vi "Simulation Initialize.vi"(0 "simulation configuration":T1={"maxTime"=5.0, "enableVisualization"=TRUE, "statechart"=path "iRobot Navigation State Machine.vi", "environment"=path "iRobot Navigation State Machine.vi", "record"=path "Simulation Record.xml", "autograde?"=TRUE, "interactive?"=FALSE, "feedback mode"=enum."debug navigation"}, 2 "Statechart display":refnum<vi>, 3 "Simulator display":refnum<vi>, 11 "Error In":errorcluster) -> (4 "simulator":T3={"configuration"={"maxTime"=5.0, "enableVisualization"=TRUE, "statechart"=path "iRobot Navigation State Machine.vi", "environment"=path "iRobot Navigation State Machine.vi", "record"=path "Simulation Record.xml", "autograde?"=TRUE, "interactive?"=FALSE, "feedback mode"=enum."debug navigation"}, "Bump Sensors"=[], "Distance Sensors"=[], "Accelerometer"=refnum, "Wall Sensor"=refnum, "Statechart\ndisplay"=refnum, "Body"=refnum, "Left Motor"=refnum, "Right Motor"=refnum, "first step?"=FALSE}, 15 "Error Out":errorcluster)   [LabVIEW 2013]
uses:
  Simulator.ctl
  <instrlib>/DC Motor Controller/HAIOL/DC Motor Controller.lvclass
  CyberSim interface/Simulation Configuration.ctl
  autograder/feedbackMode.ctl
  <vilib>/robotics/Simulator/Engine/ctl/Simulation Mode.ctl
  <vilib>/robotics/Simulator/Engine/ctl/Step Mode.ctl
  Simulation Trace Operation.ctl
  Simulation Call Statechart Operation.ctl
  <vilib>/robotics/Simulator/NI_Robotics_Simulator.lvlib
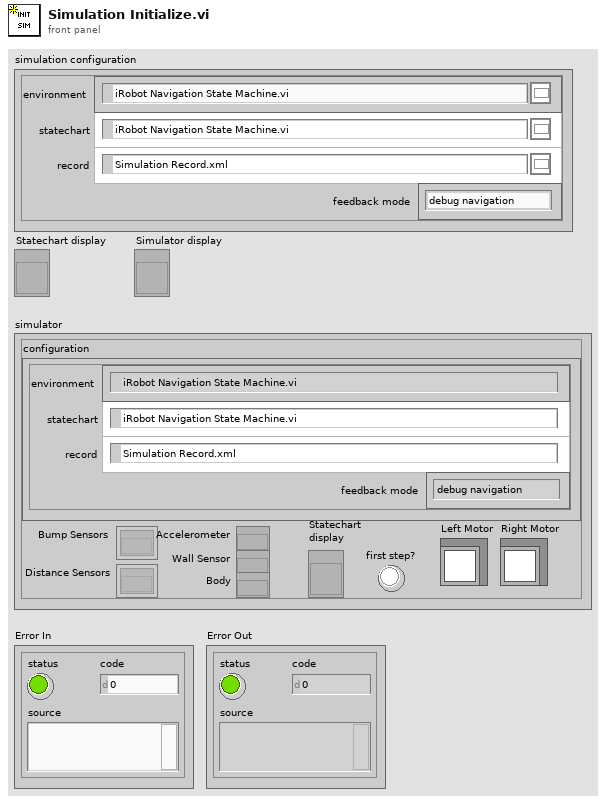
[diagram p1: front panel]
types:
  T1 = typedef "Simulation Configuration.ctl" = cluster{"maxTime":sgl, "enableVisualization":bool, "statechart":path, "environment":path, "record":path, "autograde?":bool, "interactive?":bool, "feedback mode":T2}
  T2 = typedef "feedbackMode.ctl" = enum32{"debug navigation", "debug hill climb", "autograde navigation", "autograde hill climb"}
  T3 = typedef "Simulator.ctl" = cluster{"configuration":T1, "Bump Sensors":refnum<k20>[], "Distance Sensors":refnum<k20>[], "Accelerometer":refnum<k20>, "Wall Sensor":refnum<k20>, "Statechart\ndisplay":refnum<vi>, "Body":refnum<k20>, "Left Motor":refnum<class "DC Motor Controller.lvclass">, "Right Motor":refnum<class "DC Motor Controller.lvclass">, "first step?":bool}
  T4 = typedef "Simulation Call Statechart Operation.ctl" = enum16{"Initialize", "Call Statechart", "Finalize"}
  T5 = typedef "Simulation Trace Operation.ctl" = enum16{"Initialize", "Record Trace Element", "Get Trace"}
  T6 = typedef "NI_Robotics_Simulator.lvlib/Step Mode.ctl" = u16
  T7 = typedef "NI_Robotics_Simulator.lvlib/Simulation Mode.ctl" = u16
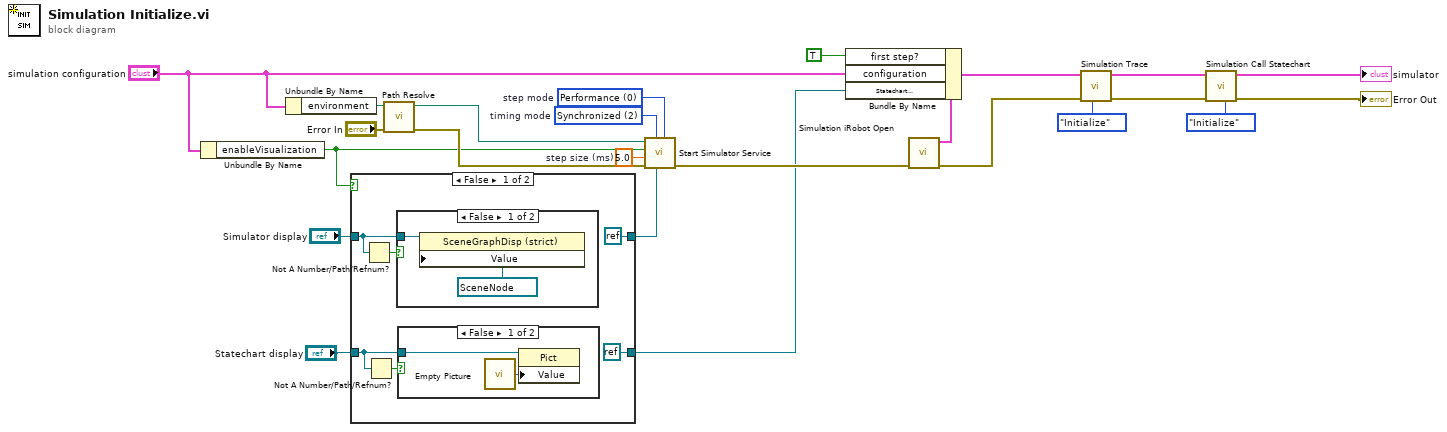
[diagram p0: block diagram]
diagram:
  w13 = 5.0  # step size (ms)
  w23 = T6 0 items=["Performance", "Accuracy"]  # step mode
  w24 = T7 2 items=["Software Real-Time", "Free Running", "Synchronized"]  # timing mode
  n1 = Unbundle By Name("simulation configuration") -> ("enableVisualization"=w9:bool)
  n2 = Unbundle By Name("simulation configuration") -> ("environment"=w17:path)
  n3 = case shown="False" w9 {
    tunnel: "Simulator display" -> [w28 w36]
    tunnel: [refnum<k0> refnum w36] -> w7
    tunnel: "Statechart display" -> [w26 w35]
    tunnel: [refnum<k0> refnum w35] -> w5
    frame False {
      n4 = Not A Number/Path/Refnum?(number/path/refnum=w28) -> (NaN/Path/Refnum?=w29:bool)
      n5 = Not A Number/Path/Refnum?(number/path/refnum=w26) -> (NaN/Path/Refnum?=w27:bool)
      n6 = case shown="False" w29 {
        tunnel: w28 -> [w34 _]
        frame False {
          n7 = property class="SceneGraphDisp (strict)"(reference=w34, "Value"=refnum<vi> refnum ("3D Picture")) -> ()  [unwired: 1 in, 2 out]
        }
        frame True {
        }
      }
      n8 = case shown="False" w27 {
        tunnel: w26 -> [w32 _]
        frame False {
          n9 = call "Empty Picture"() -> ("empty picture"=w31:picture)
          n10 = property class="Pict"(reference=w32, "Value"=w31) -> ()  [unwired: 1 in, 2 out]
        }
        frame True {
        }
      }
    }
    frame True {
    }
  }
  n11 = call "Path Resolve.vi"("Error In"="Error In", "absolute or relative path"=w17) -> ("Error Out"=w16:errorcluster, "resolved path"=w18:path)  [unwired: 8 in]
  n12 = call <vilib>:"Start Simulator Service.vi"("step mode"=w23, "3D picture refnum"=w7, "timing mode"=w24, "error in (no error)"=w16, "step size (ms)"=w13, "enable 3D visualization (T)"=w9, "manifest file"=w18) -> ("error out"=w21:errorcluster)  [unwired: 4 in]
  n13 = call "Simulation iRobot Open.vi"("error in (no error)"=w21) -> ("error out"=w14:errorcluster, "simulator"=w22:T3)  [unwired: 8 in, 1 out]
  n14 = Bundle By Name(cluster=w22, "first step?"=TRUE, "configuration"="simulation configuration", "Statechart\ndisplay"=w5) -> (w15:T3)
  n15 = call "Simulation Trace.vi"("operation"=Simulation_Trace_Operation."Initialize", "error in"=w14, "simulator"=w15) -> ("error out"=w11:errorcluster, "simulator"=w12:T3)  [unwired: 5 in, 2 out]
  n16 = call "Simulation Call Statechart.vi"("operation"=Simulation_Call_Statechart_Operation."Initialize", "error in"=w11, "simulator"=w12) -> ("error out"=→"Error Out":errorcluster, "simulator"=→"simulator":T3)  [unwired: 6 in, 1 out]
